vi "Test jsObject.vi"(8 "error in (no error)":errorcluster, 9 "Test Record (empty)":T1, 10 "Step jsObject Name (\"\")":string, 11 "Previous String (\"\")":string) -> (0 "error out":errorcluster, 2 "TEST jsObject":string, 3 "TEST definition":string)   [LabVIEW 2011]
uses:
  Test Record.ctl
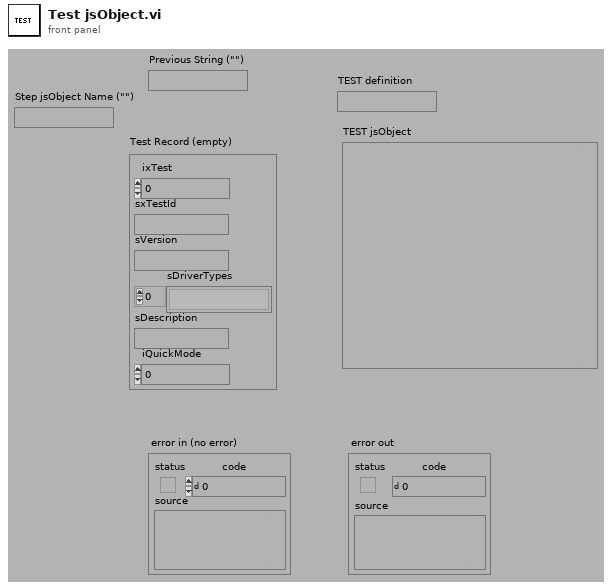
[diagram p1: front panel]
types:
  T1 = typedef "Test Record.ctl" = cluster{"ixTest":i32, "sxTestId":string, "sVersion":string, "sDriverTypes":string[], "sDescription":string, "iQuickMode":i32}
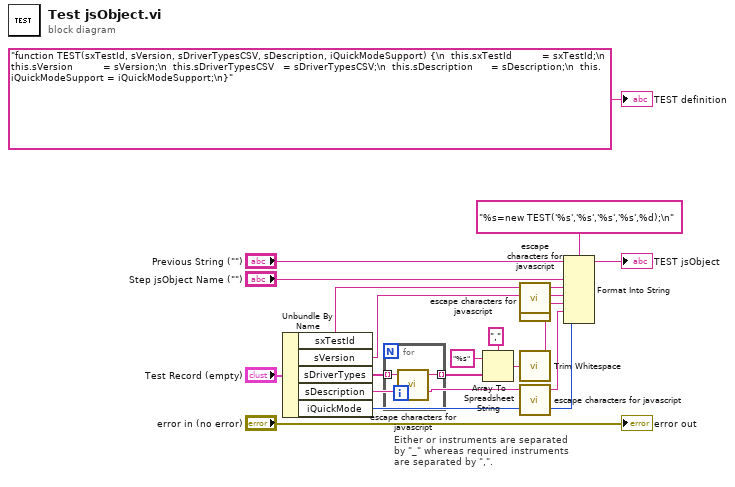
[diagram p0: block diagram]
diagram:
  # "Either or instruments are separated\nby \"_\" whereas required instruments\nare separated by \",\"."
  n1 = Unbundle By Name("Test Record (empty)") -> ("sxTestId"=w12:string, "sVersion"=w11:string, "sDriverTypes"=w7:string[], "sDescription"=w3:string, "iQuickMode"=w1:i32)
  n2 = for {
    tunnel: w7 -> [w22] mode=indexing
    tunnel: [w21] -> w6 mode=indexing
    n3 = call "escape characters for javascript.vi"("String (\"\")"=w22) -> ("escaped String"=w21:string)  [unwired: 4 out]
  }
  n4 = Array To Spreadsheet String(delimiter (Tab)=",", array=w6, 3:"%s" ("format string")) -> (spreadsheet string=w5:string)
  n5 = call "escape characters for javascript.vi"("String (\"\")"=w12) -> ("escaped String"=w14:string)  [unwired: 4 out]
  n6 = call "escape characters for javascript.vi"("String (\"\")"=w11) -> ("escaped String"=w10:string)  [unwired: 4 out]
  n7 = call <vilib>:"Trim Whitespace.vi"("string"=w5) -> ("trimmed string"=w4:string)  [unwired: 1 in]
  n8 = call "escape characters for javascript.vi"("String (\"\")"=w3) -> ("escaped String"=w2:string)  [unwired: 4 out]
  n9 = Format Into String(format string="%s=new TEST('%s','%s','%s','%s',%d);\n", initial string="Previous String (\"\")", "Step jsObject Name (\"\")", w14, w10, w4, w2, w1) -> (resulting string=→"TEST jsObject":string)  [unwired: 1 in, 1 out]
  "error out" <- "error in (no error)"
  "TEST definition" <- "function TEST(sxTestId, sVersion, sDriverTypesCSV, sDescription, iQuickModeSupport) {\n  this.sxTestId          = sxTestId;\n  this.sVersion          = sVersion;\n  this.sDriverTypesCSV   = sDriverTypesCSV;\n  this.sDescription      = sDescription;\n  this.iQuickModeSupport = iQuickModeSupport;\n}"
